vi "TREE_get active STR and active parent.vi"(8 "error in (no error)":errorcluster, 10 "Coords":T1, 11 "CtlRef":refnum<vi>) -> (0 "error out":errorcluster, 1 "Active Cell:String":string, 2 "Active Cell:Parent":string, 3 "CtlRef":refnum<vi>, 4 "Active Cell:Tag":string)   [LabVIEW 2014]
uses:
  <vilib>/Utility/miscctls.llb/LVPoint32TypeDef.ctl
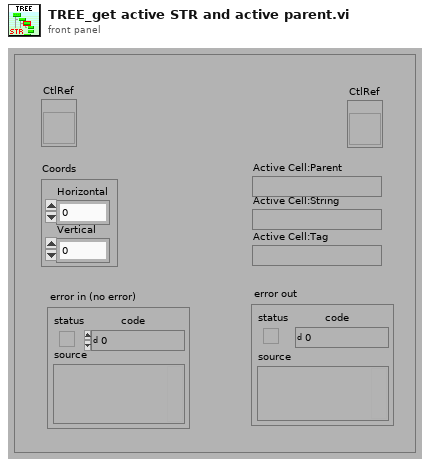
[diagram p1: front panel]
types:
  T1 = typedef "LVPoint32TypeDef.ctl" = cluster{"Horizontal":i32, "Vertical":i32}
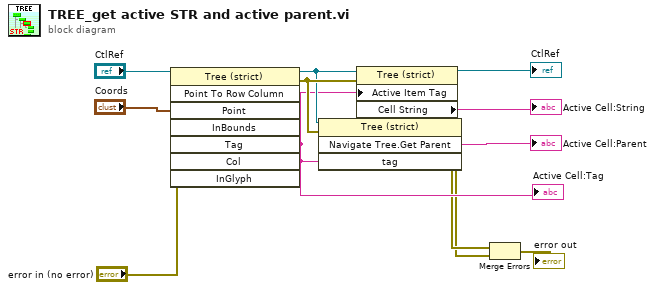
[diagram p0: block diagram]
diagram:
  n1 = invoke class="Tree (strict)" method="Point To Row Column"(reference="CtlRef", error in="error in (no error)", "Point"="Coords") -> (reference out=w9:refnum<vi>, error out=w12:errorcluster, "Tag"=w8:string)  [unwired: 5 in, 5 out]
  "Active Cell:Tag" <- w8
  n2 = invoke class="Tree (strict)" method="Navigate Tree.Get Parent"(reference=w9, error in=w12, "tag"=w8) -> (error out=w2:errorcluster, "Navigate Tree:Get Parent"=→"Active Cell:Parent":string)  [unwired: 1 in, 2 out]
  n3 = property class="Tree (strict)"(reference=w9, error in=w12, "Active Item Tag"=w8) -> (reference out=→"CtlRef":refnum<vi>, error out=w3:errorcluster, "Cell String"=→"Active Cell:String":string)
  n4 = Merge Errors(w3, w2) -> (→"error out":errorcluster)
